vi "Autoclimb.vi"(0 "Start":bool, 1 "Reset":bool, 3 "Cancel":bool, 4 "Resume":bool, 6 "DestinationLevel":T2=enum."Level 3", 7 "FrontWheelHit":bool, 10 "RaiseComplete":bool, 11 "MidWheelHit":bool) -> (12 "Front ClimberSpeed":T1, 13 "ControlRobotDrive":bool, 14 "AutoClimbState":T3, 15 "FrontClimberPosition":T2, 16 "Rear ClimberSpeed":T1, 17 "RearClimberPosition":T2, 18 "ClimbDrive":dbl format="%#_13g", 19 "RobotDrive":dbl format="%#_13g")   [LabVIEW 2019]
uses:
  TypeDefs/ClimberStates.ctl
  TypeDefs/ClimberPositions.ctl
  TypeDefs/ClimberSpeed.ctl
  ArgosLib/ArgosLib.lvlib
panel:
  in  "FinalDriveTime (ms)":u32=3000
  in  "ClimbDriveSpeed":dbl=-0.4
  in  "FastRobotDriveSpeed":dbl=-0.4
  in  "SlowRobotDriveSpeed":dbl=-0.3
  # "Inputs"
  # "Configurables"
  # "Outputs"
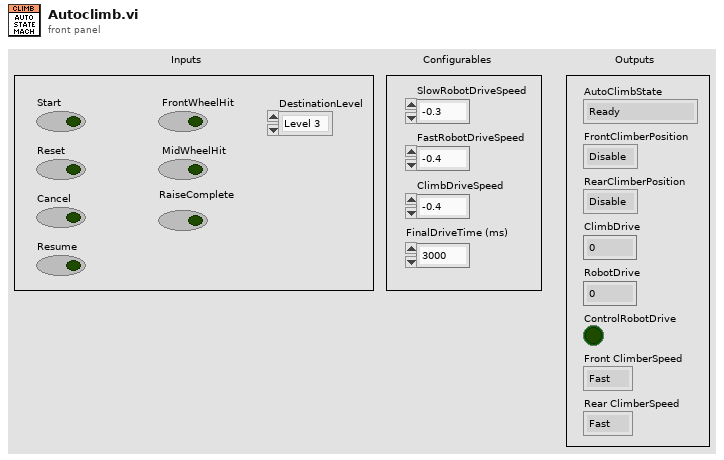
[diagram p1: front panel]
types:
  T1 = typedef "ClimberSpeed.ctl" = enum16{"Fast", "Slow"}
  T2 = typedef "ClimberPositions.ctl" = enum16{"Disable", "Floor", "Level 2", "Level 3"}
  T3 = typedef "ClimberStates.ctl" = enum16{"Ready ", "Lift Bot ", "Raised Drive", "Raise Front Sticks ", "Raise Back Sticks ", "Park ", "Cancel"}
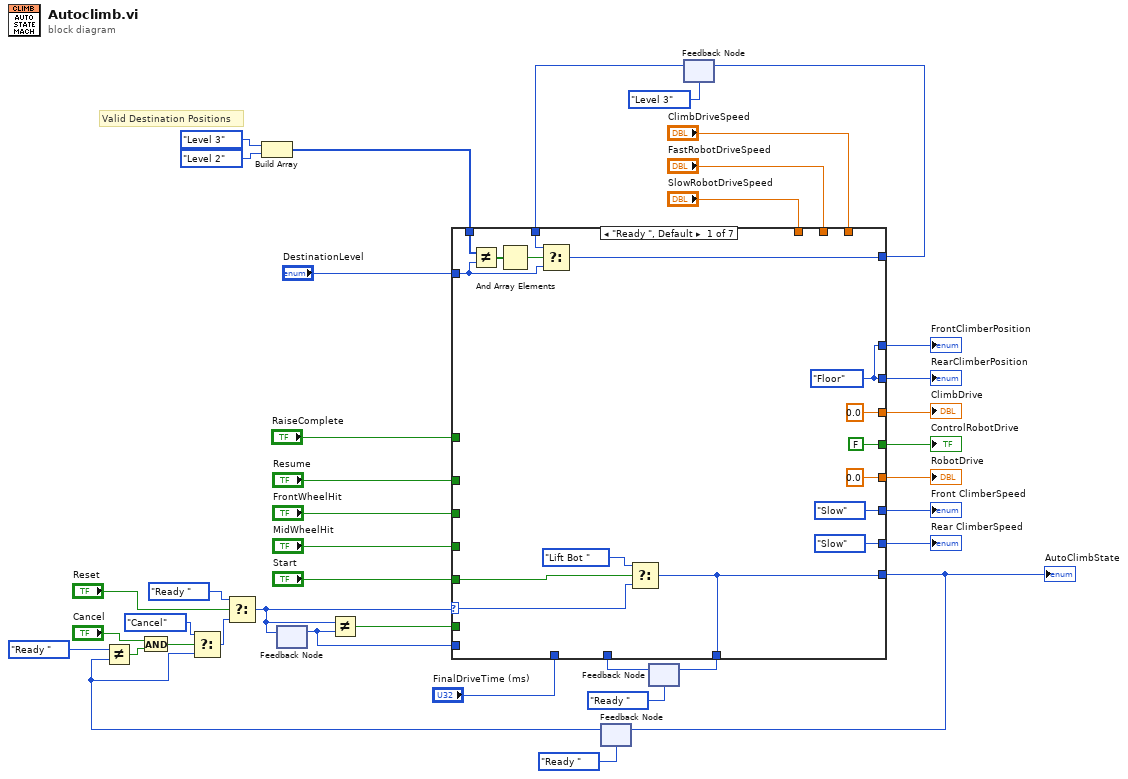
[diagram p0: block diagram]
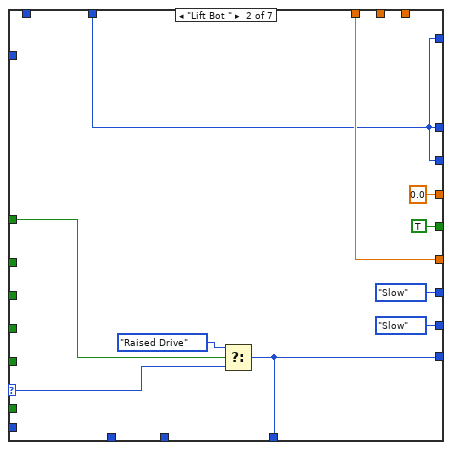
[diagram p2: hidden frame]
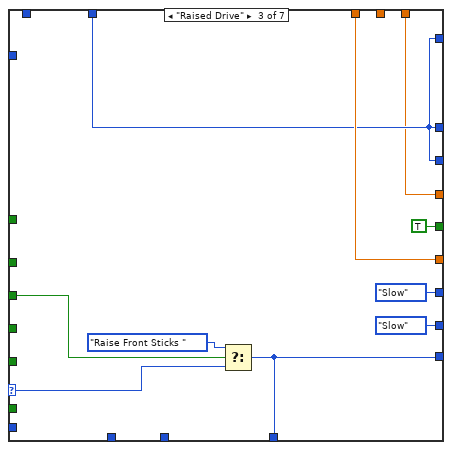
[diagram p3: hidden frame]
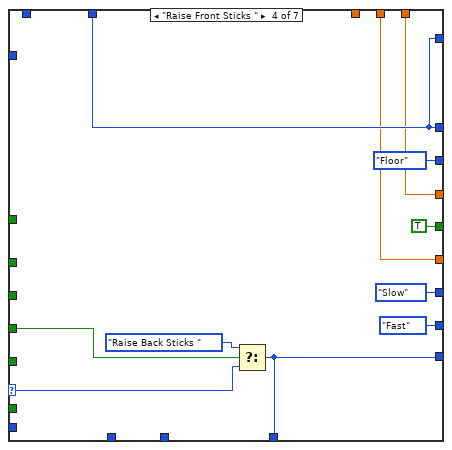
[diagram p4: hidden frame]
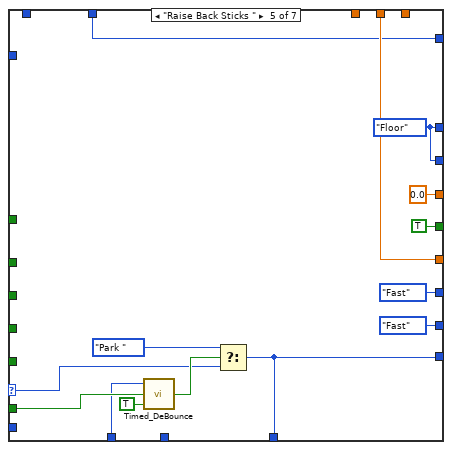
[diagram p5: hidden frame]
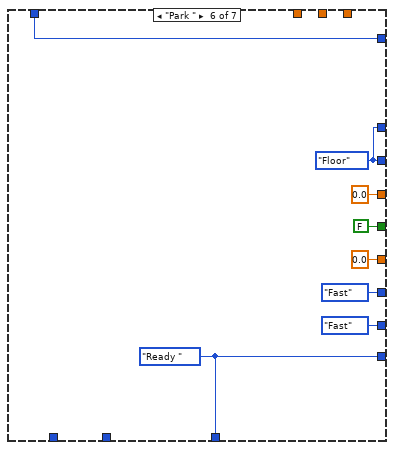
[diagram p6: hidden frame]
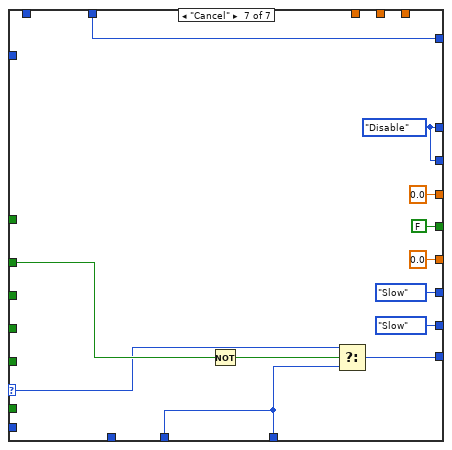
[diagram p7: hidden frame]
diagram:
  # "Valid Destination Positions"
  n1 = Build Array(ClimberPositions."Level 3" ("DestinationLevel"), ClimberPositions."Level 2" ("DestinationLevel")) -> (w27:T2[])
  n2 = feedback #1() -> (w19:T3)  [unwired: 1 in]
  n3 = feedback #2(ClimberStates."Ready " ("AutoClimbState")) -> (w12:T3)
  n4 = Not Equal?(x=ClimberStates."Ready ", y=w12) -> (x != y?=w8:bool)
  n5 = And(x="Cancel", y=w8) -> (x .and. y?=w9:bool)
  n6 = Select(t=ClimberStates."Cancel", s=w9, f=w12) -> (s? t:f=w13:T3)
  n7 = Select(t=ClimberStates."Ready ", s="Reset", f=w13) -> (s? t:f=w5:T3)
  n8 = feedback-in #1(w5) -> ()
  n9 = Not Equal?(x=w5, y=w19) -> (x != y?=w21:bool)
  n10 = feedback #3(ClimberStates."Ready " ("AutoClimbState")) -> (w16:T3)
  n11 = feedback #4(ClimberPositions."Level 3" ("DestinationLevel")) -> (w30:T2)
  n12 = case shown="\"Ready \", Default" w5 {
    selector: w5 -> [w46 w63 w73 w81 w94 _ w116]
    tunnel: [w44 w64 w74 w87 w101 w106 w121] -> w39
    tunnel: [w44 w64 w74 ClimberPositions."Floor" ("DestinationLevel") w101 w106 w121] -> w38
    tunnel: [0.0 ("ClimbDrive") 0.0 ("ClimbDriveSpeed") w70 w85 0.0 ("ClimbDriveSpeed") 0.0 ("ClimbDriveSpeed") 0.0 ("ClimbDriveSpeed")] -> w37
    tunnel: [FALSE ("ControlRobotDrive") TRUE ("ControlRobotDrive") TRUE ("ControlRobotDrive") TRUE ("ControlRobotDrive") TRUE ("ControlRobotDrive") FALSE ("ControlRobotDrive") FALSE ("ControlRobotDrive")] -> w36
    tunnel: [0.0 ("RobotDrive") w66 w76 w83 w100 0.0 ("FastRobotDriveSpeed") 0.0 ("FastRobotDriveSpeed")] -> w35
    tunnel: "DestinationLevel" -> [w50 _ _ _ _ _ _]
    tunnel: "Start" -> [w47 _ _ _ _ _ _]
    tunnel: [w48 w64 w74 w87 w92 w105 w112] -> w32
    tunnel: w30 -> [w49 w64 w74 w87 w92 w105 w112]
    tunnel: w27 -> [w53 _ _ _ _ _ _]
    tunnel: [w43 w61 w71 w79 w91 w104 w115] -> w18
    tunnel: "ClimbDriveSpeed" -> [_ _ w70 w85 _ _ _]
    tunnel: "FastRobotDriveSpeed" -> [_ _ _ w83 w100 _ _]
    tunnel: "SlowRobotDriveSpeed" -> [_ w66 w76 _ _ _ _]
    tunnel: "FrontWheelHit" -> [_ _ w69 _ _ _ _]
    tunnel: "MidWheelHit" -> [_ _ _ w82 _ _ _]
    tunnel: w21 -> [_ _ _ _ w98 _ _]
    tunnel: "FinalDriveTime (ms)" -> [_ _ _ _ w96 _ _]
    tunnel: w19 -> [_ _ _ _ _ _ _]
    tunnel: [w43 w61 w71 w79 w91 w104 w113] -> w17
    tunnel: w16 -> [_ _ _ _ _ _ w113]
    tunnel: "Resume" -> [_ _ _ _ _ _ w117]
    tunnel: "RaiseComplete" -> [_ w59 _ _ _ _ _]
    tunnel: [ClimberSpeed."Slow" ("Front ClimberSpeed") ClimberSpeed."Slow" ("Front ClimberSpeed") ClimberSpeed."Slow" ("Front ClimberSpeed") ClimberSpeed."Slow" ("Front ClimberSpeed") ClimberSpeed."Fast" ("Front ClimberSpeed") ClimberSpeed."Fast" ("Front ClimberSpeed") ClimberSpeed."Slow" ("Front ClimberSpeed")] -> w1
    tunnel: [ClimberSpeed."Slow" ("Front ClimberSpeed") ClimberSpeed."Slow" ("Front ClimberSpeed") ClimberSpeed."Slow" ("Front ClimberSpeed") ClimberSpeed."Fast" ("Front ClimberSpeed") ClimberSpeed."Fast" ("Front ClimberSpeed") ClimberSpeed."Fast" ("Front ClimberSpeed") ClimberSpeed."Slow" ("Front ClimberSpeed")] -> w2
    frame "Ready ", Default {
      w44 = ClimberPositions."Floor" ("RearClimberPosition")
      n13 = Not Equal?(x=w53, y=w50) -> (x != y?=w52:bool[])
      n14 = And Array Elements(Boolean array=w52) -> (logical AND=w51:bool)
      n15 = Select(t=w49, s=w51, f=w50) -> (s? t:f=w48:T2)
      n16 = Select(t=ClimberStates."Lift Bot ", s=w47, f=w46) -> (s? t:f=w43:T3)
    }
    frame "Lift Bot " {
      n17 = Select(t=ClimberStates."Raised Drive", s=w59, f=w63) -> (s? t:f=w61:T3)
    }
    frame "Raised Drive" {
      n18 = Select(t=ClimberStates."Raise Front Sticks ", s=w69, f=w73) -> (s? t:f=w71:T3)
    }
    frame "Raise Front Sticks " {
      n19 = Select(t=ClimberStates."Raise Back Sticks ", s=w82, f=w81) -> (s? t:f=w79:T3)
    }
    frame "Raise Back Sticks " {
      w101 = ClimberPositions."Floor" ("DestinationLevel")
      n20 = call "Timed_DeBounce.vi"("Input"=TRUE, "Reset"=w98, "Hold Time(ms)"=w96) -> ("Output"=w95:bool)
      n21 = Select(t=ClimberStates."Park ", s=w95, f=w94) -> (s? t:f=w91:T3)
    }
    frame "Park " {
      w106 = ClimberPositions."Floor" ("DestinationLevel")
      w104 = ClimberStates."Ready " ("AutoClimbState")
    }
    frame "Cancel" {
      w121 = ClimberPositions."Disable" ("DestinationLevel")
      n22 = Not(x=w117) -> (.not. x?=w114:bool)
      n23 = Select(t=w116, s=w114, f=w113) -> (s? t:f=w115:T3)
    }
  }
  "AutoClimbState" <- w18
  "FrontClimberPosition" <- w39
  "ClimbDrive" <- w37
  "RobotDrive" <- w35
  "ControlRobotDrive" <- w36
  "RearClimberPosition" <- w38
  "Front ClimberSpeed" <- w1
  "Rear ClimberSpeed" <- w2
  n24 = feedback-in #2(w18) -> ()
  n25 = feedback-in #3(w17) -> ()
  n26 = feedback-in #4(w32) -> ()
